vi "Stow Hood.vi"() -> ()   [LabVIEW 2019]
panel:
  in  "Stow Hood":bool
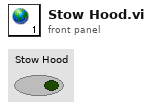
[diagram p1: front panel]
diagram:
